vi "002read_file.vi"() -> ()   [LabVIEW 2012]
panel:
  out "A波形图表":dbl[](graph)
  out "B":dbl[](array[numeric])
  out "A":dbl[](array[numeric])
  out "B波形图表":i32[](graph)
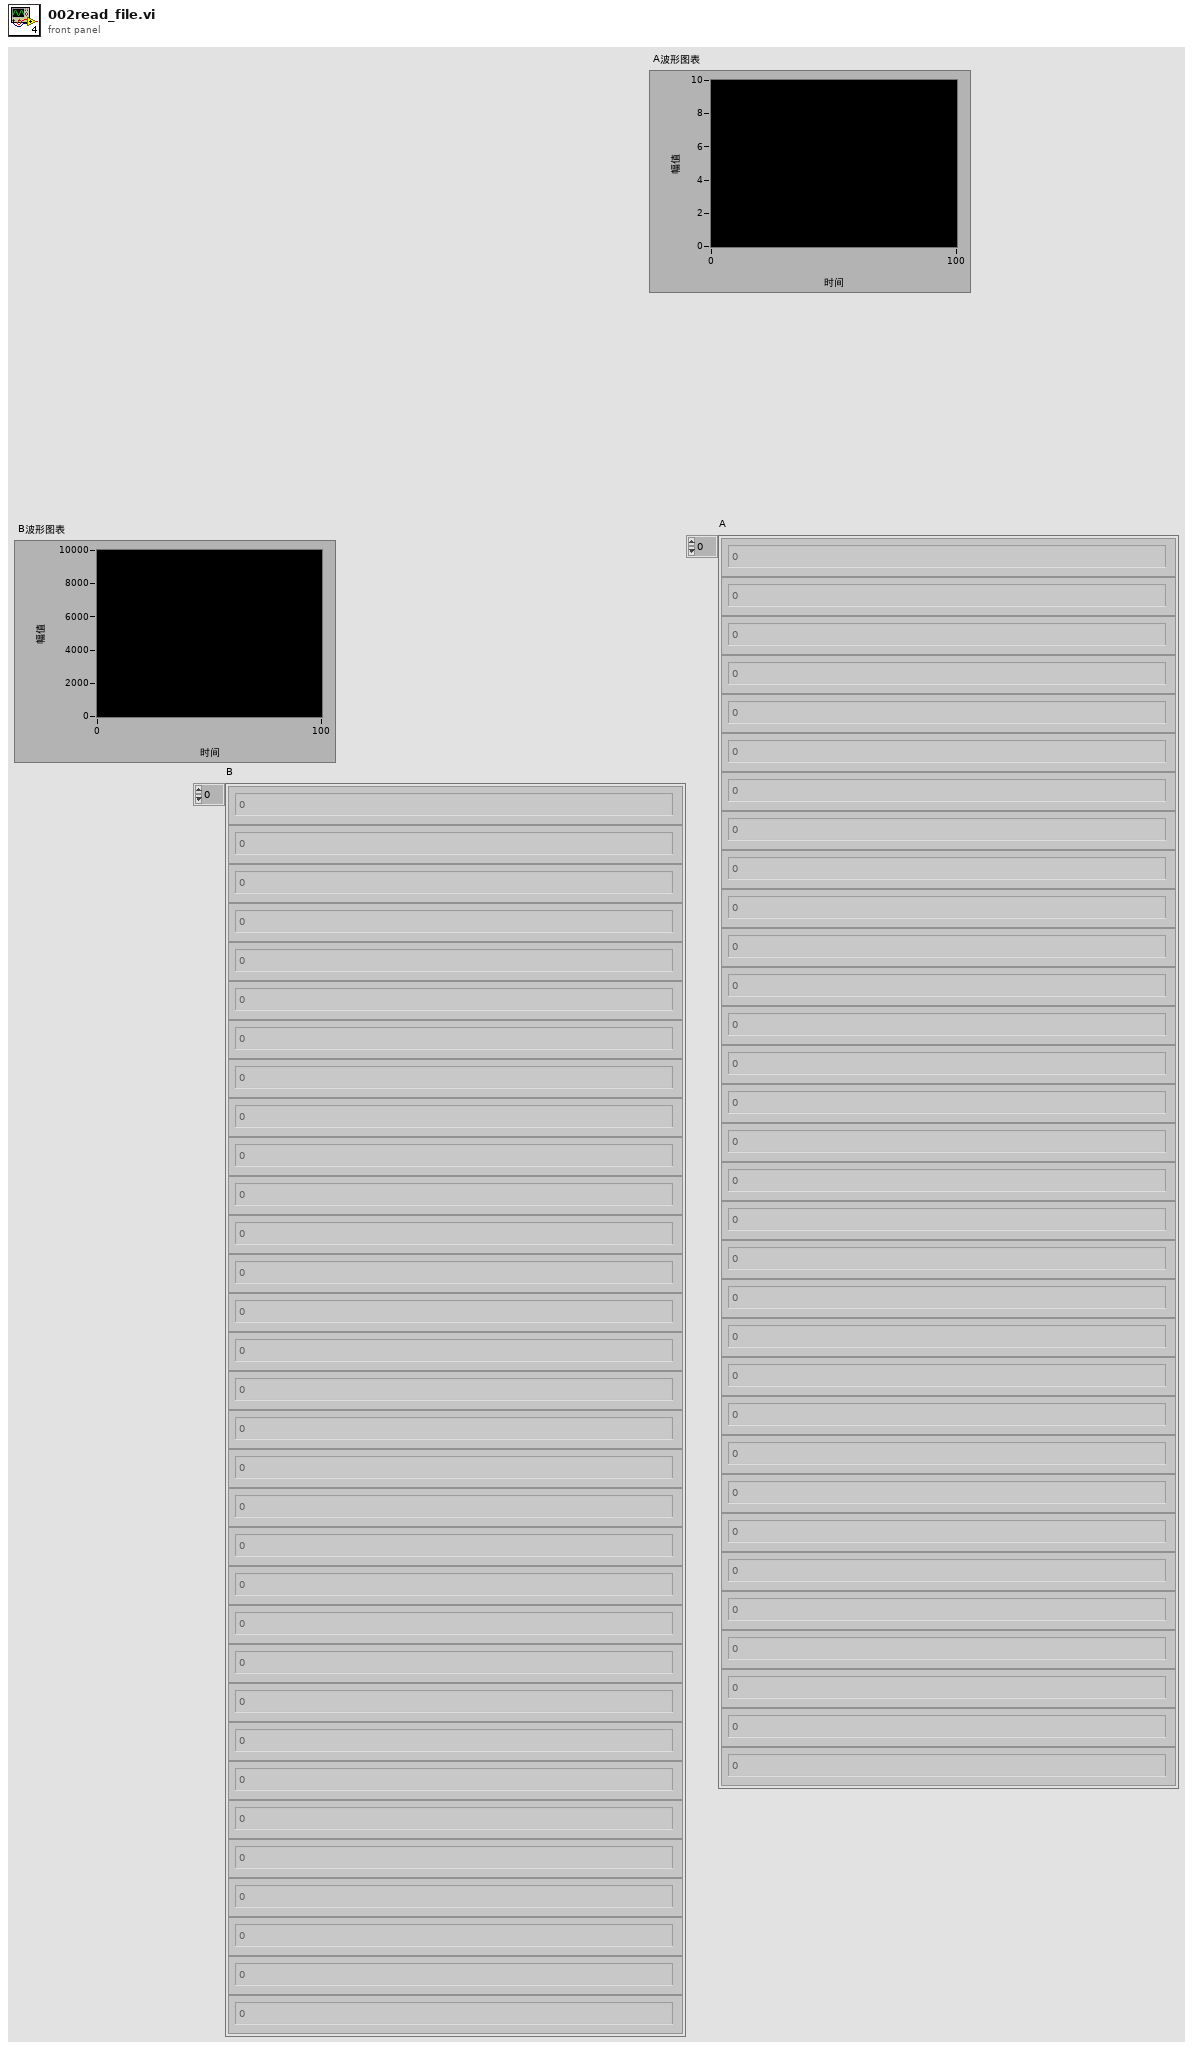
[diagram p1: front panel]
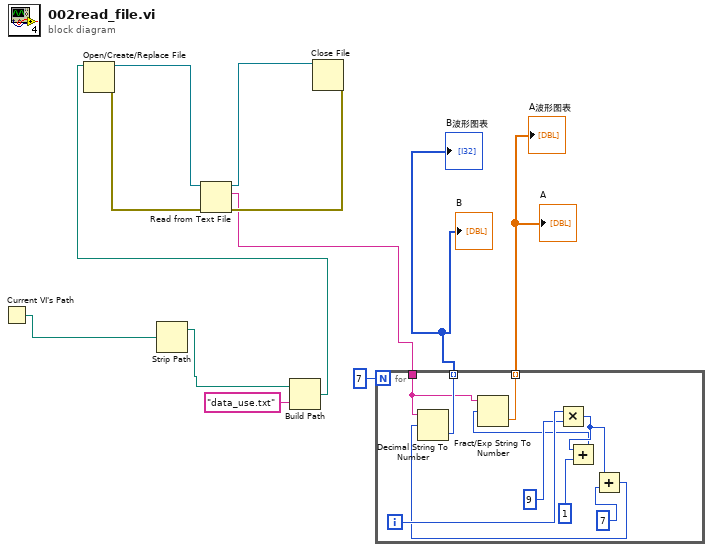
[diagram p0: block diagram]
diagram:
  n1 = Current VI's Path() -> (path=w8:path)
  n2 = Strip Path(path=w8) -> (stripped path=w6:path)  [unwired: 1 out]
  n3 = Build Path(base path=w6, name or relative path="data_use.txt" ("名称或相对路径")) -> (appended path=w5:path)
  n4 = Open/Create/Replace File(file path (use dialog)=w5) -> (refnum out=w12:refnum<file>, error out=w10:errorcluster)  [unwired: 5 in, 1 out]
  n5 = Read from Text File(file (use dialog)=w12, error in=w10) -> (refnum out=w11:refnum<file>, text=w4:string, error out=w9:errorcluster)  [unwired: 2 in, 1 out]
  n6 = Close File(refnum=w11, error in=w9) -> ()  [unwired: 2 out]
  n7 = for {
    N: 7 -> [_]
    tunnel: w4 -> [w21]
    tunnel: [w22] -> w2 mode=indexing
    tunnel: [w20] -> w1 mode=indexing
    i -> [w19]
    n8 = Multiply(x=w19, y=9) -> (x*y=w15:i32)
    n9 = Add(x=w15, y=1) -> (x+y=w14:i32)
    n10 = Fract/Exp String To Number(string=w21, offset=w14) -> (number=w20:dbl)  [unwired: 2 in, 1 out]
    n11 = Add(x=w15, y=7) -> (x+y=w13:i32)
    n12 = Decimal String To Number(string=w21, offset=w13) -> (number=w22:i32)  [unwired: 1 in, 1 out]
  }
  "B波形图表" <- w2
  "A" <- w1
  "B" <- w2
  "A波形图表" <- w1
